vi "TXD_gloval.vi"(6 "전송문자열참조":refnum<vi>, 9 "Vesa_Status":T1, 11 "SERIAL.COM_Port":refnum<visa-resource-name>) -> (1 "전송완료?":bool, 3 "전송문자열":string)   [LabVIEW 2014]
uses:
  VESA_Status.ctl
  bus_button.xctl
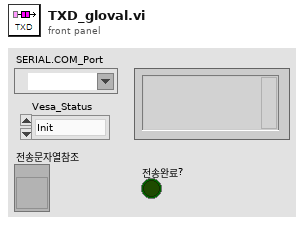
[diagram p1: front panel]
types:
  T1 = typedef "bus_button.xctl/VESA_Status.ctl" = enum16{"Init", "Wait", "Connect", "DisConnect", "Idel", "Exit"}
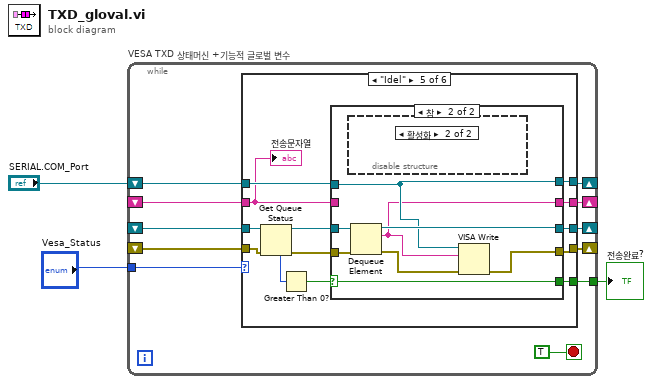
[diagram p0: block diagram]
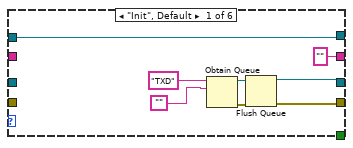
[diagram p2: hidden frame]
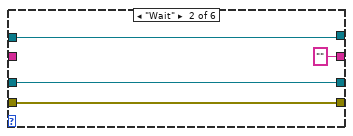
[diagram p3: hidden frame]
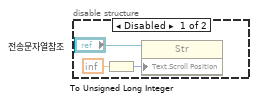
[diagram p7: hidden frame]
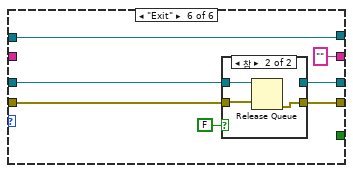
[diagram p8: hidden frame]
diagram:
  n1 = while "VESA TXD 상태머신 +기능적 글로벌 변수" {
    shift-right: [w13] -> _
    shift-left: _ -> [w11]
    shift-right: [w12] -> _
    shift-left: _ -> [w10]
    shift-right: [w9] -> _
    shift-left: _ -> [w4]
    tunnel: [w8] -> w3
    shift-right: [w6] -> _
    shift-left: "SERIAL.COM_Port" -> [w7]
    tunnel: "Vesa_Status" -> [w5]
    stop <- TRUE stop-if-true
    n2 = case shown="\"Idel\"" w5 {
      tunnel: [w18 w26 w30 w34 w40 w66] -> w13
      tunnel: [w17 w25 w29 w33 w41 w69] -> w12
      tunnel: w11 -> [_ w26 w30 w34 w47 w68]
      tunnel: w10 -> [_ w25 w29 w33 w46 w67]
      tunnel: w4 -> [_ _ w27 w31 w35 _]
      tunnel: ["" "" w27 w31 w42 ""] -> w9
      tunnel: [_ _ _ _ w39 _] -> w8
      tunnel: w7 -> [w15 w24 w28 w32 w38 w65]
      tunnel: [w15 w24 w28 w32 w37 w65] -> w6
      frame "Init", Default {
        n3 = Obtain Queue(name (unnamed)="TXD", element data type="") -> (queue out=w22:refnum<queue>, error out=w21:errorcluster)  [unwired: 3 in, 1 out]
        n4 = Flush Queue(queue=w22, error in (no error)=w21) -> (queue out=w18:refnum<queue>, error out=w17:errorcluster)  [unwired: 1 out]
      }
      frame "Wait" {
      }
      frame "Connect" {
      }
      frame "DisConnect" {
      }
      frame "Idel" {
        n5 = Get Queue Status(queue=w47, error in (no error)=w46) -> (queue out=w44:refnum<queue>, error out=w43:errorcluster, # elements in queue=w45:i32)  [unwired: 1 in, 5 out]
        n6 = Greater Than 0?(x=w45) -> (x > 0?=w36:bool)
        n7 = case shown="참" w36 {
          selector: w36 -> [_ w54]
          tunnel: w44 -> [w50 w59]
          tunnel: w43 -> [w49 w58]
          tunnel: w35 -> [w51 _]
          tunnel: [w51 w52] -> w42
          tunnel: [w49 w56] -> w41
          tunnel: w38 -> [w48 w53]
          tunnel: [w50 w55] -> w40
          tunnel: [_ w54] -> w39
          tunnel: [w48 w53] -> w37
          frame False {
          }
          frame True {
            n8 = disable-structure shown="활성화" {
              frame Disabled {
                n9 = To Unsigned Long Integer(number=inf) -> (unsigned 32bit integer=w61:u32)
                n10 = property class="Str"(reference="전송문자열참조", "Text.Scroll Position"=w61) -> ()  [unwired: 1 in, 2 out]
              }
              frame Enabled {
              }
            }
            n11 = Dequeue Element(queue=w59, error in (no error)=w58) -> (queue out=w55:refnum<queue>, element=w52:string, error out=w57:errorcluster)  [unwired: 1 in, 1 out]
            n12 = VISA Write(VISA resource name=w53, write buffer=w52, error in (no error)=w57) -> (error out=w56:errorcluster)  [unwired: 2 out]
          }
        }
        "전송문자열" <- w35
      }
      frame "Exit" {
        n13 = case shown="참" FALSE {
          tunnel: [w71 w72] -> w69
          tunnel: w68 -> [w70 w74]
          tunnel: w67 -> [w71 w73]
          tunnel: [w70 _] -> w66
          frame False {
          }
          frame True {
            n14 = Release Queue(queue=w74, error in (no error)=w73) -> (error out=w72:errorcluster)  [unwired: 1 in, 2 out]
          }
        }
      }
    }
  }
  "전송완료?" <- w3
